vi "Get Value as Variant.vi"(8 "error in (no error)":errorcluster, 11 "CVT_DBL in":refnum<class "CVT_DBL.lvclass">) -> (0 "error out":errorcluster, 2 "data":variant, 3 "CVT_DBL out":refnum<class "CVT_DBL.lvclass">)   [LabVIEW 2024, in "Current Value Table.lvlib" / "CVT_DBL.lvclass"]
uses:
  CVT_DBL.lvclass
  CVT_DBL.lvclass/CVT_DBL.ctl
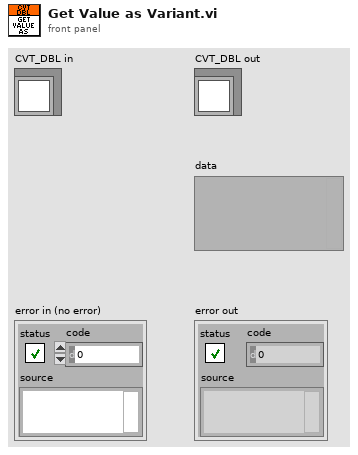
[diagram p1: front panel]
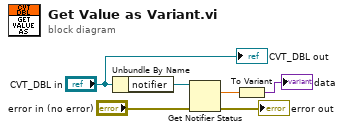
[diagram p0: block diagram]
diagram:
  n1 = Unbundle By Name("CVT_DBL in") -> ("notifier"=w5:refnum<notifier>)
  n2 = Get Notifier Status(notifier=w5, error in (no error)="error in (no error)") -> (current notification=w4:dbl, error out=→"error out":errorcluster)  [unwired: 3 out]
  n3 = To Variant(anything=w4) -> (Variant=→"data":variant)
  "CVT_DBL out" <- "CVT_DBL in"
